vi "Do Action.vi"(4 "error in (no error)":errorcluster, 6 "Array in":refnum<class>[](array[class]), 7 "Act_Append Many in":refnum<class "Act_Append Many.lvclass">) -> (0 "error out":errorcluster, 2 "Array out":refnum<class>[](array[class]), 3 "Act_Append Many out":refnum<class "Act_Append Many.lvclass">)   [LabVIEW 2014, in "Act_Append Many.lvclass"]
uses:
  Act_Append Many.lvclass
  Act_Append Many.lvclass/Act_Append Many.ctl
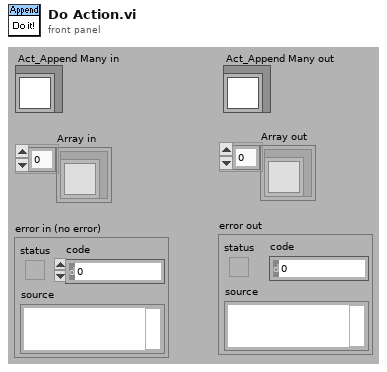
[diagram p1: front panel]
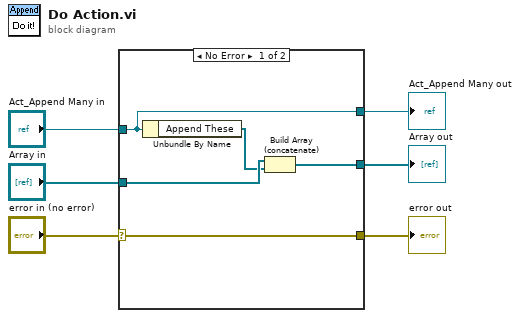
[diagram p0: block diagram]
diagram:
  n1 = case shown="No Error" "error in (no error)" {
    selector: "error in (no error)" -> [w7 w12]
    tunnel: "Array in" -> [w11 w13]
    tunnel: "Act_Append Many in" -> [w8 w14]
    tunnel: [w9 w13] -> w3
    tunnel: [w8 w14] -> w2
    tunnel: [w7 w12] -> w1
    frame No Error {
      n2 = Unbundle By Name(w8) -> ("Append These"=w10:refnum<class>[])
      n3 = Build Array (concatenate)(w11, w10) -> (w9:refnum<class>[])
    }
    frame Error {
    }
  }
  "error out" <- w1
  "Array out" <- w3
  "Act_Append Many out" <- w2
